vi "OFDM-SIM1导频.vi"(1 "输入的OFDM符号":cdb[](array[numeric])) -> (0 "OFDM-IM output":cdb[](array[numeric]))   [LabVIEW 2018]
uses:
  <vilib>/Analysis/1siggen.llb/Ramp Pattern by Samples.vi
  <vilib>/Analysis/NI_AALBase.lvlib
panel:
  out "加导频后":cdb[](array[numeric])
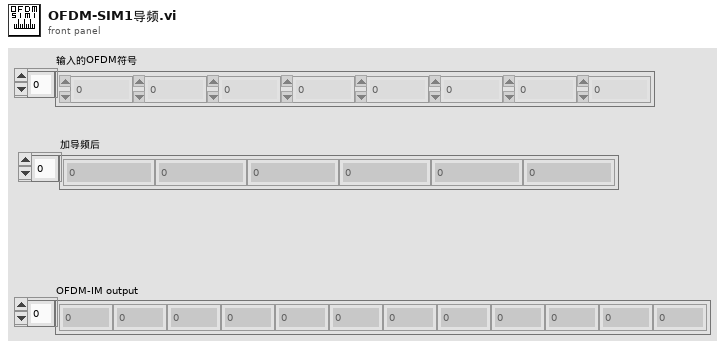
[diagram p1: front panel]
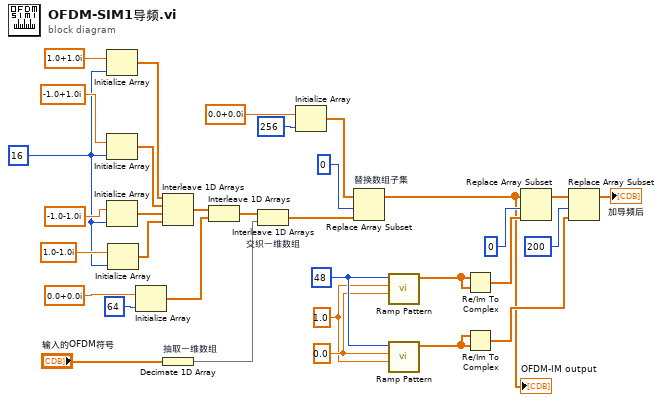
[diagram p0: block diagram]
diagram:
  w1 = 16
  w18 = 1.0
  w19 = 0.0
  w20 = 48
  n1 = Initialize Array(cdb 1.0+1.0i, w1) -> (w8:cdb[])
  n2 = Initialize Array(cdb -1.0+1.0i, w1) -> (w5:cdb[])
  n3 = Initialize Array(cdb -1.0-1.0i, w1) -> (w6:cdb[])
  n4 = Initialize Array(cdb 1.0-1.0i, w1) -> (w7:cdb[])
  n5 = Initialize Array(cdb 0.0+0.0i, 64) -> (w11:cdb[])
  n6 = Interleave 1D Arrays(w8, w5, w6, w7) -> (w9:cdb[])
  n7 = Decimate 1D Array "抽取一维数组"("输入的OFDM符号") -> (w30:cdb[])
  n8 = Interleave 1D Arrays(w9, w11) -> (w10:cdb[])
  n9 = Interleave 1D Arrays "交织一维数组"(w10, w30) -> (w17:cdb[])
  n10 = Initialize Array(cdb 0.0+0.0i ("元素"), 256 ("维数大小")) -> (w29:cdb[])
  n11 = Replace Array Subset "替换数组子集"(array=w29, new element=w17, index=0 ("索引")) -> (w15:cdb[])
  "OFDM-IM output" <- w15
  n12 = call-poly <vilib>:"Ramp Pattern.vi"("start"=w19, "end"=w18, "samples"=w20) -> ("Ramp Pattern"=w27:dbl[])  [unwired: 7 in, 1 out]
  n13 = call-poly <vilib>:"Ramp Pattern.vi"("start"=w18, "end"=w19, "samples"=w20) -> ("Ramp Pattern"=w23:dbl[])  [unwired: 7 in, 1 out]
  n14 = Re/Im To Complex(1:w27, 2:w27) -> (0:w26:cdb[])
  n15 = Re/Im To Complex(1:w23, 2:w23) -> (0:w22:cdb[])
  n16 = Replace Array Subset(array=w15, new element=w26, index=0) -> (w21:cdb[])
  n17 = Replace Array Subset(array=w21, new element=w22, index=200) -> (→"加导频后":cdb[])
